vi "HomingTest.vi"() -> ()   [LabVIEW 2011]
uses:
  <vilib>/Analysis/NI_AALBase.lvlib
panel:
  out "Valeur du home":T1(graph)={"X Values"=[50.6, 51.8, 53.0, 54.2, 55.4, 56.6, 57.8, 59.0, 60.2, 61.4], "Histogram: h(x)"=[4, 6, 12, 22, 11, 20, 13, 12, 8, 2]}
  out "Array":dbl[](array[numeric])=[57.0, 53.0, 54.0, 52.0, 53.0, 54.0, 54.0, 55.0, 54.0, 54.0, 55.0, 54.0, 52.0, 53.0, 54.0, 52.0, 53.0, 54.0, 57.0, 53.0, 51.0, 59.0, 53.0, 51.0, 52.0, 55.0, 54.0, 52.0, 55.0, 54.0, 54.0, 60.0, 54.0, 55.0, 55.0, 54.0, 54.0, 58.0, 56.0, 50.0, 51.0, 54.0, 57.0, 53.0, 56.0, 52.0, 53.0, 56.0, 53.0, 58.0, 54.0, 55.0, 56.0, 54.0, 55.0, 53.0, 54.0, 55.0, 56.0, 57.0, 55.0, 53.0, 54.0, 58.0, 53.0, 54.0, 60.0, 59.0, 54.0, 58.0, 59.0, 57.0, 62.0, 56.0, 54.0, 55.0, 56.0, 57.0, 58.0, 59.0, 59.0, 58.0, 56.0, 60.0, 58.0, 61.0, 60.0, 58.0, 59.0, 57.0, 58.0, 56.0, 57.0, 58.0, 59.0, 57.0, 58.0, 59.0, 60.0, 60.0, 59.0, 57.0, 58.0, 59.0, 57.0, 58.0, 59.0, 60.0, 60.0, 59.0]
  out "Homed":bool=TRUE
  out "VRN":refnum<visa-resource-name>="COM10"
  in  "STOP":bool
  in  "GO":bool
  in  "BackDistance":i32=10000
  in  "Accel_B":dbl=10000.0
  in  "Fast_B":dbl=10000.0
  in  "Slow_B":dbl=1.0
  in  "Accel_A":dbl=20000.0
  in  "Fast_A":dbl=30000.0
  in  "Slow_A":dbl=1.0
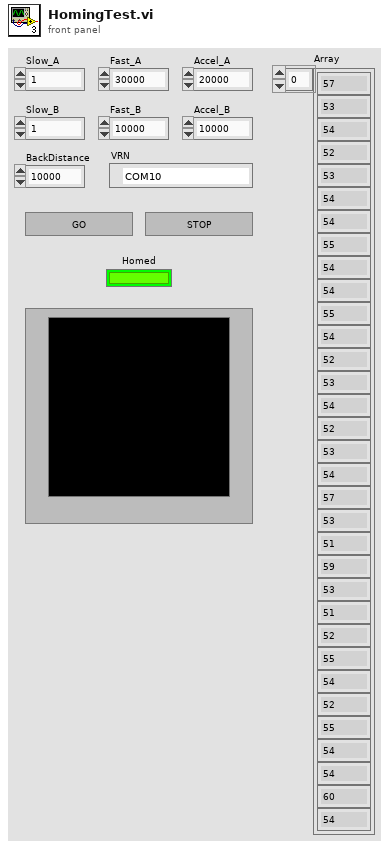
[diagram p1: front panel]
types:
  T1 = cluster{"X Values":dbl[], "Histogram: h(x)":i32[]}
  T2 = enum8{"Enabled", "Disabled", "Disabled and Grayed Out"}
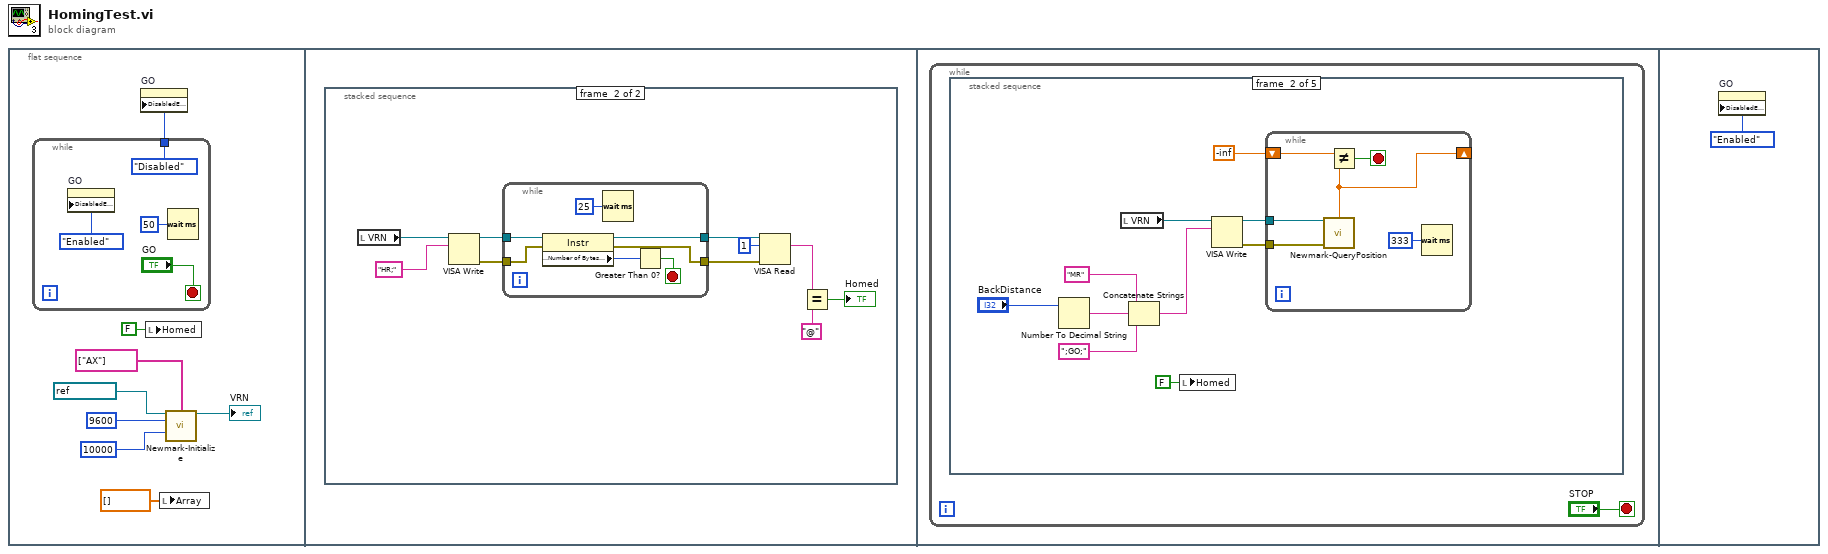
[diagram p0: block diagram]
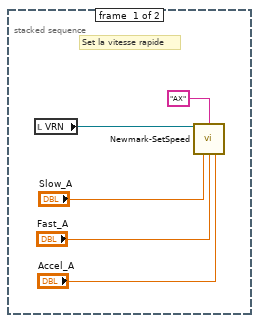
[diagram p2: hidden frame]
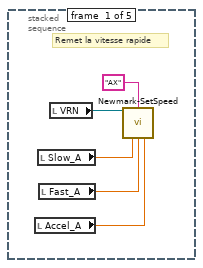
[diagram p3: hidden frame]
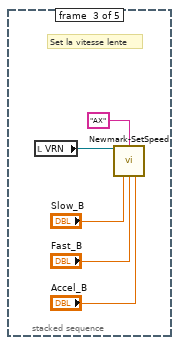
[diagram p4: hidden frame]
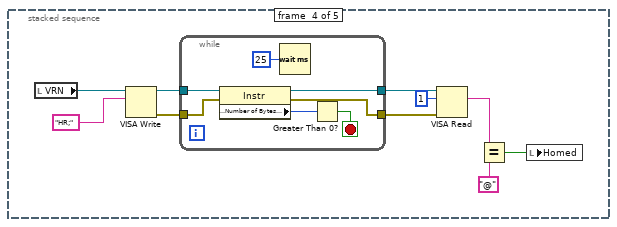
[diagram p5: hidden frame]
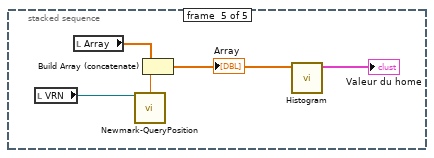
[diagram p6: hidden frame]
diagram:
  n1 = flat-sequence {
    frame #0 {
      n2 = while {
        tunnel: [T2."Disabled" ("Disabled")] -> w8
        stop <- "GO" stop-if-true
        n3 = property on="GO" class="Bool"("DisabledEnum"=T2."Enabled" ("Disabled")) -> ()  [unwired: 2 in, 2 out]
        n4 = Wait (ms)(milliseconds to wait=u32 50) -> ()  [unwired: 1 out]
      }
      n5 = property on="GO" class="Bool"("DisabledEnum"=w8) -> ()  [unwired: 2 in, 2 out]
      n6 = local write "Homed"(FALSE ("Homed")) -> ()
      n7 = local write "Array"(dbl[] [] ("Array")) -> ()
      n8 = call "Newmark-Initialize.vi"("VISA resource name"=refnum<visa-resource-name> "COM10", "ActiveStages"=string[] ["AX"], "baud rate"=u32 9600, "Timeout"=u32 10000) -> ("VISA resource name out"=→"VRN":refnum<visa-resource-name>)  [unwired: 10 in, 1 out]
    }
    frame #1 {
      n9 = stacked-sequence {
        frame #0 {
          # "Set la vitesse rapide"
          n10 = local read "VRN"() -> (w16:refnum<visa-resource-name>)
          n11 = call "Newmark-SetSpeed.vi"("Table VRN"=w16, "StageTAG"="AX", "Vitesse Lente"="Slow_A", "Vitesse Rapide"="Fast_A", "Accélération"="Accel_A") -> ()  [unwired: 8 in, 3 out]
        }
        frame #1 {
          n12 = local read "VRN"() -> (w27:refnum<visa-resource-name>)
          n13 = VISA Write(VISA resource name=w27, write buffer="HR;") -> (VISA resource name out=w25:refnum<visa-resource-name>, error out=w24:errorcluster)  [unwired: 1 in, 1 out]
          n14 = while {
            tunnel: w25 -> [w34]
            tunnel: w24 -> [w33]
            tunnel: [w29] -> w23
            tunnel: [w28] -> w22
            stop <- w31 stop-if-true
            n15 = property class="Instr"(reference=w34, error in=w33) -> (reference out=w29:refnum<visa-resource-name>, error out=w28:errorcluster, "Serial Settings:Number of Bytes at Serial Port"=w32:u32)
            n16 = Wait (ms)(milliseconds to wait=u32 25) -> ()  [unwired: 1 out]
            n17 = Greater Than 0?(x=w32) -> (x > 0?=w31:bool)
          }
          n18 = VISA Read(VISA resource name=w23, byte count=u32 1, error in (no error)=w22) -> (read buffer=w20:string)  [unwired: 3 out]
          n19 = Equal?(x=w20, y="@") -> (x = y?=→"Homed":bool)
        }
      }
    }
    frame #2 {
      n20 = while {
        stop <- "STOP" stop-if-true
        n21 = stacked-sequence {
          frame #0 {
            # "Remet la vitesse rapide"
            n22 = local read "Accel_A"() -> (w36:dbl)
            n23 = local read "Slow_A"() -> (w38:dbl)
            n24 = local read "Fast_A"() -> (w37:dbl)
            n25 = local read "VRN"() -> (w40:refnum<visa-resource-name>)
            n26 = call "Newmark-SetSpeed.vi"("Table VRN"=w40, "StageTAG"="AX", "Vitesse Lente"=w38, "Vitesse Rapide"=w37, "Accélération"=w36) -> ()  [unwired: 8 in, 3 out]
          }
          frame #1 {
            n27 = Number To Decimal String(number="BackDistance") -> (decimal integer string=w43:string)  [unwired: 1 in]
            n28 = local read "VRN"() -> (w48:refnum<visa-resource-name>)
            n29 = Concatenate Strings("MR", w43, ";GO;") -> (w42:string)
            n30 = local write "Homed"(FALSE ("Homed")) -> ()
            n31 = VISA Write(VISA resource name=w48, write buffer=w42) -> (VISA resource name out=w49:refnum<visa-resource-name>, error out=w50:errorcluster)  [unwired: 1 in, 1 out]
            n32 = while {
              tunnel: w49 -> [w56]
              tunnel: w50 -> [w55]
              shift-right: [w52] -> _
              shift-left: -inf -> [w53]
              stop <- w54 stop-if-true
              n33 = call "Newmark-QueryPosition.vi"("Table VRN IN"=w56, "Error IN"=w55) -> ("X Axis"=w52:dbl)  [unwired: 7 in, 6 out]
              n34 = Not Equal?(x=w53, y=w52) -> (x != y?=w54:bool)
              n35 = Wait (ms)(milliseconds to wait=u32 333) -> ()  [unwired: 1 out]
            }
          }
          frame #2 {
            # "Set la vitesse lente"
            n36 = local read "VRN"() -> (w61:refnum<visa-resource-name>)
            n37 = call "Newmark-SetSpeed.vi"("Table VRN"=w61, "StageTAG"="AX", "Vitesse Lente"="Slow_B", "Vitesse Rapide"="Fast_B", "Accélération"="Accel_B") -> ()  [unwired: 8 in, 3 out]
          }
          frame #3 {
            n38 = local read "VRN"() -> (w63:refnum<visa-resource-name>)
            n39 = VISA Write(VISA resource name=w63, write buffer="HR;") -> (VISA resource name out=w65:refnum<visa-resource-name>, error out=w66:errorcluster)  [unwired: 1 in, 1 out]
            n40 = while {
              tunnel: w65 -> [w78]
              tunnel: w66 -> [w77]
              tunnel: [w73] -> w67
              tunnel: [w72] -> w68
              stop <- w75 stop-if-true
              n41 = property class="Instr"(reference=w78, error in=w77) -> (reference out=w73:refnum<visa-resource-name>, error out=w72:errorcluster, "Serial Settings:Number of Bytes at Serial Port"=w76:u32)
              n42 = Wait (ms)(milliseconds to wait=u32 25) -> ()  [unwired: 1 out]
              n43 = Greater Than 0?(x=w76) -> (x > 0?=w75:bool)
            }
            n44 = VISA Read(VISA resource name=w67, byte count=u32 1, error in (no error)=w68) -> (read buffer=w70:string)  [unwired: 3 out]
            n45 = Equal?(x=w70, y="@") -> (x = y?=w62:bool)
            n46 = local write "Homed"(w62) -> ()
          }
          frame #4 {
            n47 = local read "VRN"() -> (w83:refnum<visa-resource-name>)
            n48 = local read "Array"() -> (w82:dbl[])
            n49 = call "Newmark-QueryPosition.vi"("Table VRN IN"=w83) -> ("X Axis"=w81:dbl)  [unwired: 8 in, 6 out]
            n50 = Build Array (concatenate)(w82, w81) -> (w80:dbl[])
            "Array" <- w80
            n51 = call <vilib>:"Histogram.vi"("X"=w80) -> ("Histogram Graph"=→"Valeur du home":T1)  [unwired: 7 in, 3 out]
          }
        }
      }
    }
    frame #3 {
      n52 = property on="GO" class="Bool"("DisabledEnum"=T2."Enabled" ("Disabled")) -> ()  [unwired: 2 in, 2 out]
    }
  }
